vi "Disable & Enable.vi"(8 "error in (no error)":errorcluster, 9 "Disabled?":bool, 11 "Control Ref Array":refnum<vi>[](array[refnum])) -> (0 "error out":errorcluster)   [LabVIEW 2020, in "3D Plot.lvclass"]
uses:
  <vilib>/Math Plots/3D Math Plots/3D Plot/3D Plot/3D Plot.lvclass
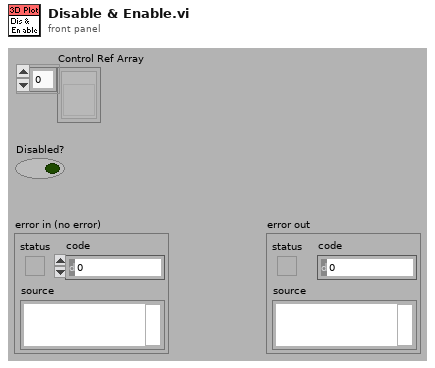
[diagram p1: front panel]
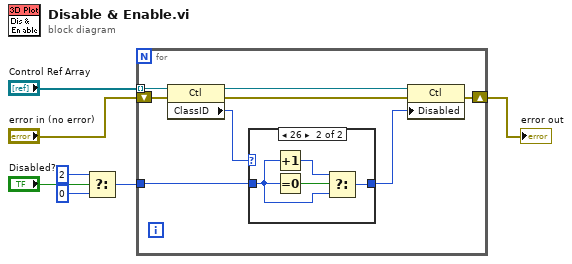
[diagram p0: block diagram]
diagram:
  n1 = Select(t=u8 2 ("Disabled"), s="Disabled?", f=u8 0 ("Disabled")) -> (s? t:f=w7:u8)
  n2 = for {
    tunnel: "Control Ref Array" -> [w15] mode=indexing
    tunnel: w7 -> [w10]
    shift-right: [w14] -> w1
    shift-left: "error in (no error)" -> [w9]
    n3 = property class="Ctl"(reference=w15, error in=w9) -> (reference out=w13:refnum<vi>, error out=w8:errorcluster, "ClassID"=w12:u32)
    n4 = case shown="26" w12 {
      tunnel: [w16 w17] -> w11
      tunnel: w10 -> [w16 w18]
      frame Default {
      }
      frame 26 {
        n5 = Increment(x=w18) -> (x+1=w19:u8)
        n6 = Equal To 0?(x=w18) -> (x = 0?=w20:bool)
        n7 = Select(t=w19, s=w20, f=w18) -> (s? t:f=w17:u8)
      }
    }
    n8 = property class="Ctl"(reference=w13, error in=w8, "Disabled"=w11) -> (error out=w14:errorcluster)  [unwired: 1 out]
  }
  "error out" <- w1
